vi "select array index value.vi"(7 "Sort by which item":T1, 8 "error in":errorcluster, 11 "cycle results cluster":T2) -> (0 "error out":errorcluster, 2 "value that will be sorted":i32, 4 "string array values":string[](array[string]))   [LabVIEW 2016]
doc: "determines which column is going to be used to sort the cycle results"
uses:
  controls/cycle results control.ctl
  controls/cycle sort control.ctl
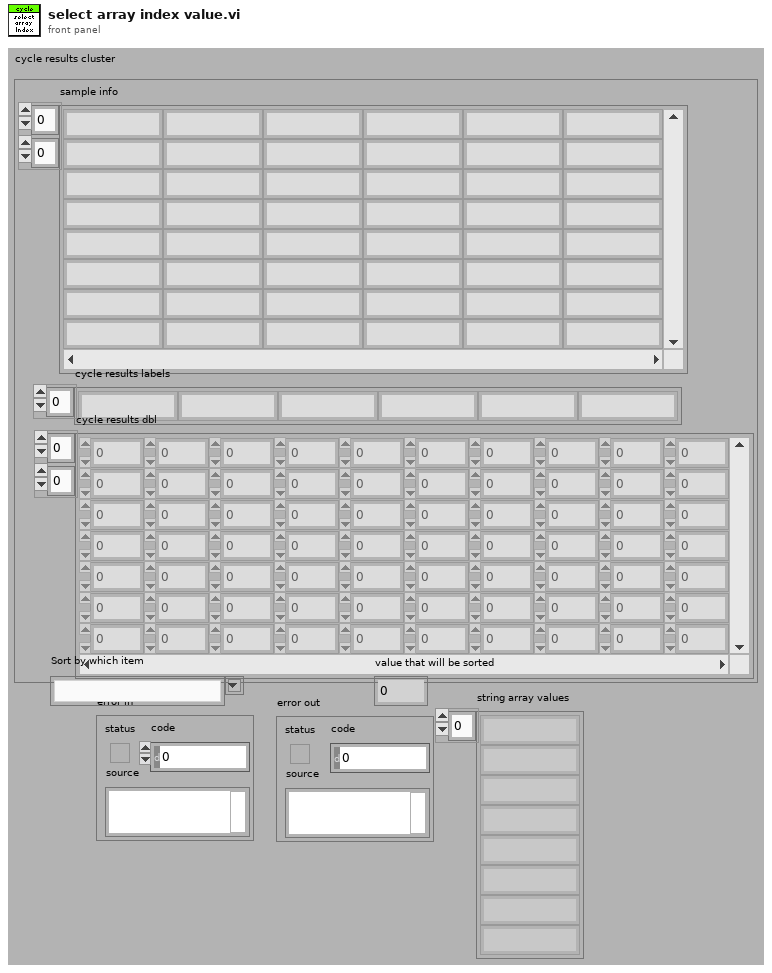
[diagram p1: front panel]
types:
  T1 = typedef "cycle sort control.ctl" = string
  T2 = typedef "cycle results control.ctl" = cluster{"sample info":string[][], "cycle results labels":string[], "cycle results dbl":dbl[][]}
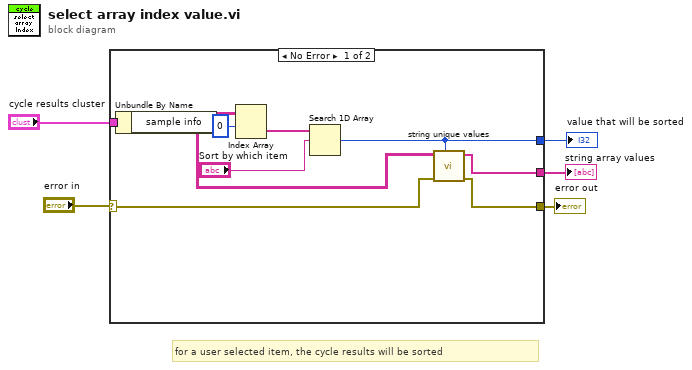
[diagram p0: block diagram]
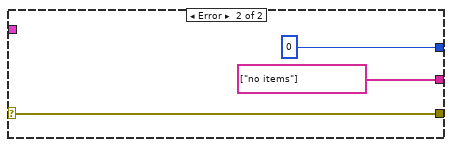
[diagram p2: hidden frame]
diagram:
  # "for a user selected item, the cycle results will be sorted"
  n1 = case shown="No Error" "error in" {
    selector: "error in" -> [w9 w17]
    tunnel: "cycle results cluster" -> [w14 _]
    tunnel: [w6 0 ("index of element")] -> w4
    tunnel: [w8 w17] -> w2
    tunnel: [w7 string[] ["no items"] ("string array values")] -> w1
    frame No Error {
      n2 = Unbundle By Name(w14) -> ("sample info"=w10:string[][])
      n3 = Index Array(array=w10, index (row)=0) -> (element=w12:string[])  [unwired: 1 in]
      n4 = Search 1D Array(1D array=w12, element="Sort by which item") -> (index of element=w6:i32)  [unwired: 1 in]
      n5 = call "string unique values.vi"("index of element"=w6, "error in"=w9, "sample info"=w10) -> ("error out"=w8:errorcluster, "string array values"=w7:string[])  [unwired: 7 in]
    }
    frame Error {
    }
  }
  "error out" <- w2
  "value that will be sorted" <- w4
  "string array values" <- w1
